vi "Read.vi"(8 "error in (no error)":errorcluster, 9 "timeout in ms (-1)":i32=-1, 11 "queue out":T1) -> (0 "error out":errorcluster, 1 "Data":variant, 2 "Message":string, 4 "timeout?":bool, 5 "Sender":string)   [LabVIEW 2016, in "System.lvlib"]
uses:
  System.lvlib
  Controls/Control_Queue Reference.ctl
  Controls/Control_Message Data.ctl
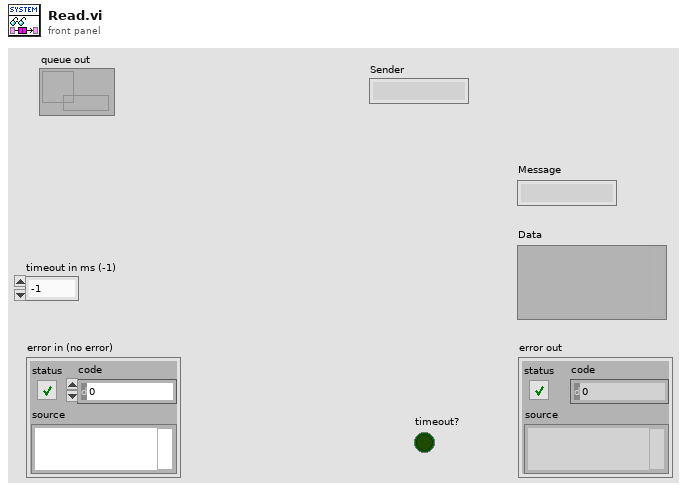
[diagram p1: front panel]
types:
  T1 = typedef "System.lvlib/Control_Queue Reference.ctl" = refnum<queue>
  T2 = typedef "System.lvlib/Control_Message Data.ctl" = cluster{"Message":string, "Data":variant, "Sender":string}
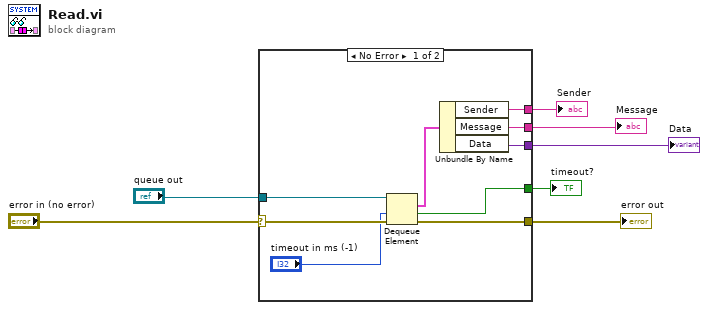
[diagram p0: block diagram]
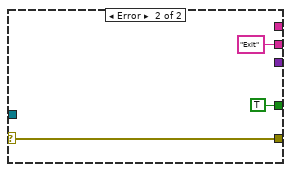
[diagram p2: hidden frame]
diagram:
  n1 = case shown="No Error" "error in (no error)" {
    selector: "error in (no error)" -> [w15 w19]
    tunnel: "queue out" -> [w16 _]
    tunnel: [w13 w19] -> w3
    tunnel: [w11 "Exit" ("Message")] -> w7
    tunnel: [w10 _] -> w6
    tunnel: [w9 TRUE ("timed out?")] -> w5
    tunnel: [w8 _] -> w1
    frame No Error {
      n2 = Dequeue Element(queue=w16, timeout in ms (-1)="timeout in ms (-1)", error in (no error)=w15) -> (element=w12:T2, timed out?=w9:bool, error out=w13:errorcluster)  [unwired: 1 out]
      n3 = Unbundle By Name(w12) -> ("Sender"=w8:string, "Message"=w11:string, "Data"=w10:variant)
    }
    frame Error {
    }
  }
  "Data" <- w6
  "Message" <- w7
  "timeout?" <- w5
  "error out" <- w3
  "Sender" <- w1
